vi "Check Freq Cal Pass.vi"(8 "error in (no error)":errorcluster) -> (0 "error out":errorcluster, 3 "function return":bool)   [LabVIEW 2013, in "QCAWLAN_DLL.lvlib"]
doc: "QCA_DLL_Export bool CheckFreqCalPass();"
uses:
  QCAWLAN_DLL.lvlib
  QCAWLAN_DLL.dll
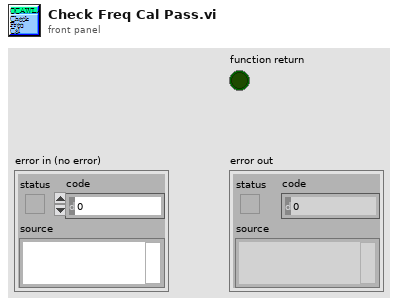
[diagram p1: front panel]
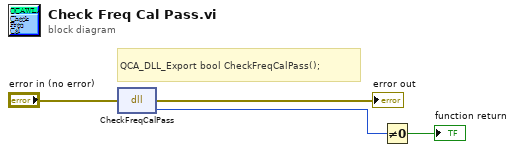
[diagram p0: block diagram]
diagram:
  # "QCA_DLL_Export bool CheckFreqCalPass();"
  n1 = dll-call lib="C:/Users/dave_yao/Desktop/Hitron/QCA9984 WLAN_LV2013/user.lib/QCAWLAN_DLL/QCAWLAN_DLL.*" fn="CheckFreqCalPass"(error in="error in (no error)") -> (error out=→"error out":errorcluster, w3:u8)  [unwired: 2 in, 1 out]
  n2 = Not Equal To 0?(x=w3) -> (x != 0?=→"function return":bool)
